vi "Framework.Get Transceiver Loader.vi"(11 "Framework in":refnum<class "Framework.lvclass">) -> (2 "Transceiver Loader":refnum<class "DSF.Engine.Transceiver Loader.lvclass">, 3 "Framework out":refnum<class "Framework.lvclass">)   [LabVIEW 2017, in "DSF.Engine.lvlib" / "Framework.lvclass"]
uses:
  Framework.lvclass
  Transceiver/DSF.Engine.Transceiver Loader.lvclass
  Framework.lvclass/Framework.ctl
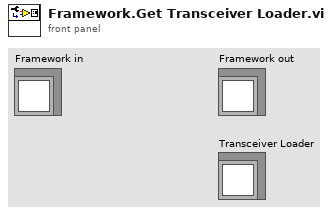
[diagram p1: front panel]
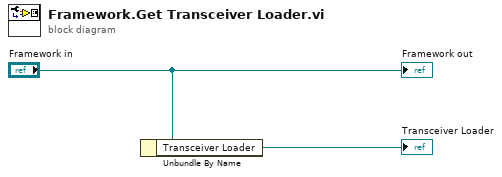
[diagram p0: block diagram]
diagram:
  n1 = Unbundle By Name("Framework in") -> ("Transceiver Loader"=→"Transceiver Loader":refnum<class "DSF.Engine.Transceiver Loader.lvclass">)
  "Framework out" <- "Framework in"
